vi "Read.vi"(8 "error in (no error)":errorcluster, 10 "Reset Counter":bool, 11 "Encoder Ref In":T2) -> (0 "error out":errorcluster, 1 "Overflow?":bool, 2 "Counter Value":i32, 3 "Encoder Ref Out":T2, 4 "Counter Direction":T1)   [LabVIEW 2021, in "Encoder.lvlib"]
doc: "Reads the value of the encoder tick counter, the last direction of the tick counter, and whether the counter wraps around."
uses:
  <vilib>/myRIO/Instrument Drivers/Onboard IO/Encoder/Encoder.lvlib
  <vilib>/myRIO/Instrument Drivers/Onboard IO/Encoder/typedefs/Encoder Reference.ctl
  <vilib>/myRIO/Common/Instrument Driver Framework/Utilities/typedefs/myRIO Generic Hardware Reference.ctl
  <vilib>/myRIO/Common/Instrument Driver Framework/Utilities/typedefs/Hardware Version Enum.ctl
  <vilib>/myRIO/Common/Instrument Driver Framework/Utilities/typedefs/myRIO v1.0 Reference.ctl
  <vilib>/myRIO/Common/Instrument Driver Framework/Utilities/typedefs/Generic FPGA Reference.ctl
  <vilib>/myRIO/Common/Instrument Driver Framework/myRIO v1.0/Encoder/typedefs/Encoder Channels Enum.ctl
  <vilib>/myRIO/Common/Instrument Driver Framework/myRIO v1.0/Encoder/typedefs/Encoder Count Direction Enum.ctl
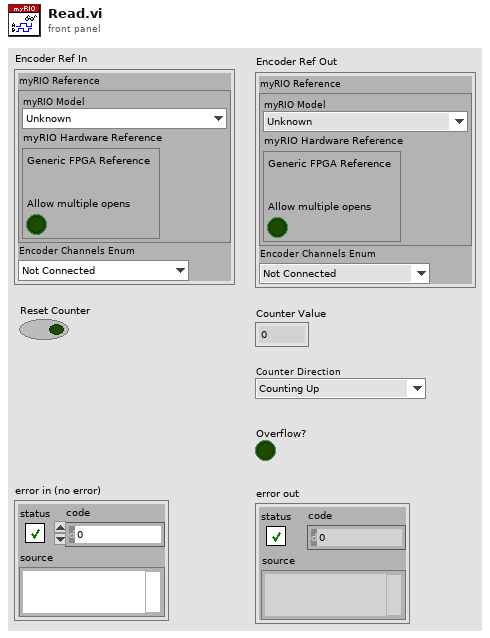
[diagram p1: front panel]
types:
  T1 = typedef "Encoder Count Direction Enum.ctl" = enum16{"Counting Up", "Counting Down"}
  T2 = typedef "Encoder.lvlib/Encoder Reference.ctl" = cluster{"myRIO Reference":T3, "Encoder Channels Enum":T7}
  T3 = typedef "myRIO Generic Hardware Reference.ctl" = cluster{"myRIO Model":T4, "myRIO Hardware Reference":T5}
  T4 = typedef "Hardware Version Enum.ctl" = enum16{"Unknown", "myRIO-1900", "myRIO-1950", "roboRIO", "NI ELVIS RIO CM", "ELVIS III"}
  T5 = typedef "myRIO v1.0 Reference.ctl" = cluster{"Generic FPGA Reference":T6, "Allow multiple opens":bool}
  T6 = typedef "Generic FPGA Reference.ctl" = refnum<k20>
  T7 = typedef "Encoder Channels Enum.ctl" = enum16{"Not Connected", "C/ENC0", "C/ENC1", "A/ENC", "A/ENC0", "A/ENC1", "A/ENC2", "A/ENC3", "A/ENC4", "A/ENC5", "A/ENC6", "A/ENC7", "A/ENC8", "A/ENC9", "B/ENC", "B/ENC0", "B/ENC1", "B/ENC2", "B/ENC3", "B/ENC4", "B/ENC5", "B/ENC6", "B/ENC7", "B/ENC8", "B/ENC9", "DIO/ENC0", "DIO/ENC1", "DIO/ENC2", "DIO/ENC3", "DIO/ENC4"}
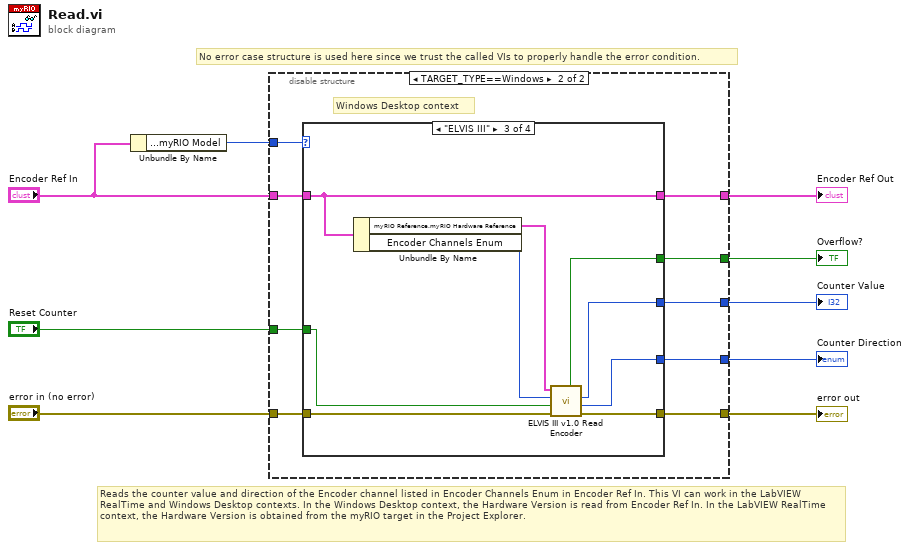
[diagram p0: block diagram]
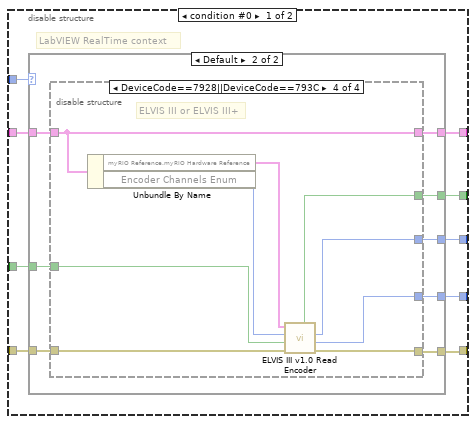
[diagram p2: hidden frame]
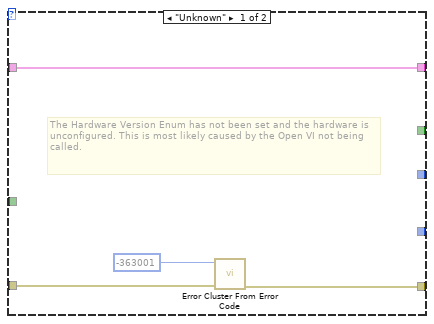
[diagram p3: hidden frame]
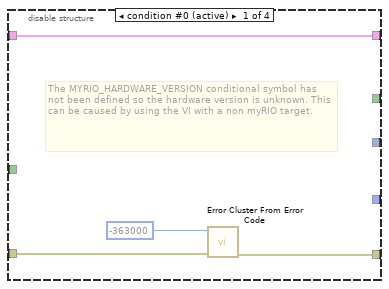
[diagram p4: hidden frame]
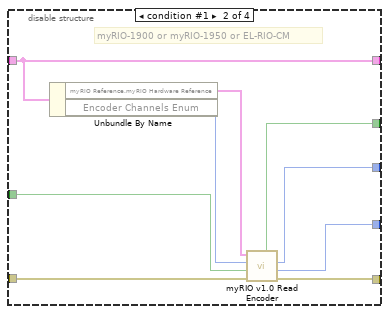
[diagram p5: hidden frame]
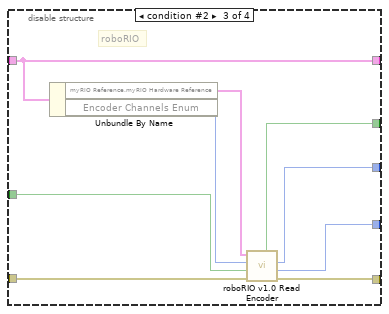
[diagram p6: hidden frame]
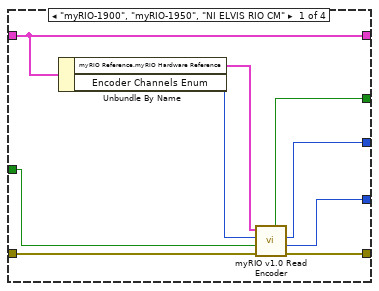
[diagram p7: hidden frame]
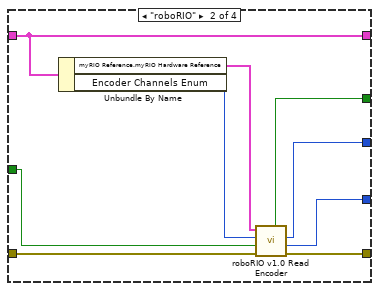
[diagram p8: hidden frame]
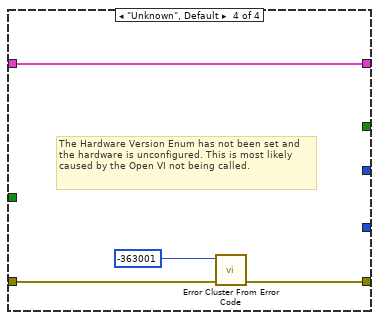
[diagram p9: hidden frame]
diagram:
  # "No error case structure is used here since we trust the called VIs to properly handle the error condition."
  # "Reads the counter value and direction of the Encoder channel listed in Encoder Channels Enum in Encoder Ref In. This VI can work in the LabVIEW RealTime and Windows Desktop contexts. In the Windows Desktop context, the Hardware Version is read from Encoder Ref In. In the LabVIEW RealTime context, the Hardware Version is obtained from the myRIO target in the Project Explorer."
  n1 = Unbundle By Name("Encoder Ref In") -> ("myRIO Reference.myRIO Model"=w1:T4)
  n2 = disable-structure shown="TARGET_TYPE==Windows" {
    disable-tunnel: [w18 w70] -> w6
    disable-tunnel: "Encoder Ref In" -> [w17 w67]
    disable-tunnel: "error in (no error)" -> [w16 w69]
    disable-tunnel: [w15 w68] -> w7
    disable-tunnel: w1 -> [w14 w66]
    disable-tunnel: "Reset Counter" -> [w13 w65]
    disable-tunnel: [w12 w64] -> w4
    disable-tunnel: [w11 w63] -> w3
    disable-tunnel: [w10 w62] -> w2
    frame condition #0 {
      # "LabVIEW RealTime context"
      n3 = case shown="Default" w14 {
        tunnel: [w21 w30] -> w18
        tunnel: w17 -> [w19 w29]
        tunnel: w16 -> [w20 w28]
        tunnel: [w19 w27] -> w15
        tunnel: w13 -> [_ w26]
        tunnel: [_ w25] -> w12
        tunnel: [_ w24] -> w11
        tunnel: [_ w23] -> w10
        frame "Unknown" {
          # "The Hardware Version Enum has not been set and the hardware is unconfigured. This is most likely caused by the Open VI not being called."
          n4 = call <vilib>:"Error Cluster From Error Code.vi"("error in (no error)"=w20, "error code (0)"=-363001) -> ("error out"=w21:errorcluster)  [unwired: 7 in]
        }
        frame Default {
          n5 = disable-structure shown="DeviceCode==7928||DeviceCode==793C" {
            disable-tunnel: w29 -> [w31 w42 w51 w59]
            disable-tunnel: [w34 w40 w49 w56] -> w30
            disable-tunnel: w28 -> [w32 w41 w50 w57]
            disable-tunnel: [w31 w42 w51 w59] -> w27
            disable-tunnel: w26 -> [_ w38 w47 w58]
            disable-tunnel: [_ w37 w46 w54] -> w25
            disable-tunnel: [_ w36 w45 w55] -> w24
            disable-tunnel: [_ w35 w44 w53] -> w23
            frame condition #0 (active) {
              # "The MYRIO_HARDWARE_VERSION conditional symbol has not been defined so the hardware version is unknown. This can be caused by using the VI with a non myRIO target."
              n6 = call <vilib>:"Error Cluster From Error Code.vi"("error in (no error)"=w32, "error code (0)"=-363000) -> ("error out"=w34:errorcluster)  [unwired: 7 in]
            }
            frame condition #1 {
              # "myRIO-1900 or myRIO-1950 or EL-RIO-CM"
              n7 = Unbundle By Name(w42) -> ("myRIO Reference.myRIO Hardware Reference"=w43:T5, "Encoder Channels Enum"=w39:T7)
              n8 = call <vilib>:"myRIO v1.0 Read Encoder.vi"("error in (no error)"=w41, "Reset Counter"=w38, "Channel"=w39, "myRIO Ref In"=w43) -> ("error out"=w40:errorcluster, "Counter Direction"=w36:T1, "Counter Value"=w37:i32, "Overflow?"=w35:bool)  [unwired: 3 in, 1 out]
            }
            frame condition #2 {
              # "roboRIO"
              n9 = Unbundle By Name(w51) -> ("myRIO Reference.myRIO Hardware Reference"=w52:T5, "Encoder Channels Enum"=w48:T7)
              n10 = call <vilib>:"roboRIO v1.0 Read Encoder.vi"("error in (no error)"=w50, "Reset Counter"=w47, "Channel"=w48, "myRIO Ref In"=w52) -> ("error out"=w49:errorcluster, "Counter Direction"=w45:T1, "Counter Value"=w46:i32, "Overflow?"=w44:bool)  [unwired: 3 in, 1 out]
            }
            frame condition #3 {
              # "ELVIS III or ELVIS III+"
              n11 = Unbundle By Name(w59) -> ("myRIO Reference.myRIO Hardware Reference"=w61:T5, "Encoder Channels Enum"=w60:T7)
              n12 = call <vilib>:"ELVIS III v1.0 Read Encoder.vi"("error in (no error)"=w57, "Reset Counter"=w58, "Channel"=w60, "myRIO Ref In"=w61) -> ("error out"=w56:errorcluster, "Counter Direction"=w55:T1, "Counter Value"=w54:i32, "Overflow?"=w53:bool)  [unwired: 3 in, 1 out]
            }
          }
        }
      }
    }
    frame condition #1 (active) {
      # "Windows Desktop context"
      n13 = case shown="\"ELVIS III\"" w66 {
        tunnel: [w77 w86 w91 w101] -> w70
        tunnel: w67 -> [w78 w87 w95 w98]
        tunnel: w69 -> [w76 w85 w90 w99]
        tunnel: [w78 w87 w95 w98] -> w68
        tunnel: w65 -> [w74 w83 w89 _]
        tunnel: [w73 w82 w93 _] -> w64
        tunnel: [w72 w81 w92 _] -> w63
        tunnel: [w71 w80 w94 _] -> w62
        frame "myRIO-1900", "myRIO-1950", "NI ELVIS RIO CM" {
          n14 = Unbundle By Name(w78) -> ("myRIO Reference.myRIO Hardware Reference"=w79:T5, "Encoder Channels Enum"=w75:T7)
          n15 = call <vilib>:"myRIO v1.0 Read Encoder.vi"("error in (no error)"=w76, "Reset Counter"=w74, "Channel"=w75, "myRIO Ref In"=w79) -> ("error out"=w77:errorcluster, "Counter Direction"=w72:T1, "Counter Value"=w73:i32, "Overflow?"=w71:bool)  [unwired: 3 in, 1 out]
        }
        frame "roboRIO" {
          n16 = Unbundle By Name(w87) -> ("myRIO Reference.myRIO Hardware Reference"=w88:T5, "Encoder Channels Enum"=w84:T7)
          n17 = call <vilib>:"roboRIO v1.0 Read Encoder.vi"("error in (no error)"=w85, "Reset Counter"=w83, "Channel"=w84, "myRIO Ref In"=w88) -> ("error out"=w86:errorcluster, "Counter Direction"=w81:T1, "Counter Value"=w82:i32, "Overflow?"=w80:bool)  [unwired: 3 in, 1 out]
        }
        frame "ELVIS III" {
          n18 = Unbundle By Name(w95) -> ("myRIO Reference.myRIO Hardware Reference"=w97:T5, "Encoder Channels Enum"=w96:T7)
          n19 = call <vilib>:"ELVIS III v1.0 Read Encoder.vi"("error in (no error)"=w90, "Reset Counter"=w89, "Channel"=w96, "myRIO Ref In"=w97) -> ("error out"=w91:errorcluster, "Counter Direction"=w92:T1, "Counter Value"=w93:i32, "Overflow?"=w94:bool)  [unwired: 3 in, 1 out]
        }
        frame "Unknown", Default {
          # "The Hardware Version Enum has not been set and the hardware is unconfigured. This is most likely caused by the Open VI not being called."
          n20 = call <vilib>:"Error Cluster From Error Code.vi"("error in (no error)"=w99, "error code (0)"=-363001) -> ("error out"=w101:errorcluster)  [unwired: 7 in]
        }
      }
    }
  }
  "Encoder Ref Out" <- w7
  "error out" <- w6
  "Counter Value" <- w4
  "Counter Direction" <- w3
  "Overflow?" <- w2
